vi "observacao.vi"() -> ()   [LabVIEW 2018, in "Shared_160.lvlib"] (continued)
                      }
                      frame True {
                        # "stop"
                      }
                    }
                  }
                  frame 3 {
                    w3458 = "TENTE NOVAMENTE" ("SYSTEM MESSAGES")
                    # "Trata Timeout"
                    n2721 = call "TickTimeout.vi"() -> ("msTick"=w3459:u32)  [unwired: 2 in, 2 out]
                    n2722 = call "Monta_Mensagem.vi"("Mensagem"=w3458) -> ()  [unwired: 2 in]
                    n2723 = call "Salva_systems_messages.vi"("Mensagem"=w3458) -> ()  [unwired: 5 in]
                    n2724 = local write "Timeout PROT"(w3459) -> ()
                  }
                  frame 4 {
                    w3462 = u16 1 items=["ZERO", "AH", "DEC", "TUBO", "CUP"] ("Controlador")
                    w3467 = u16 2 items=["ZERO", "AH", "DEC", "TUBO", "CUP"] ("Controlador")
                    # "Para os motores"
                    n2725 = call "Monta Comando.vi"("Comando"="PARAR", "Dispositivo"="PROG", "Controlador"=w3462) -> ()  [unwired: 2 in, 5 out]
                    n2726 = call "Monta Comando.vi"("Comando"="PARAR", "Dispositivo"="PROG", "Controlador"=w3467) -> ()  [unwired: 2 in, 5 out]
                  }
                  frame 5 {
                    # "SAÍDA"
                  }
                }
                n2727 = local write "M_PROT"(w3430) -> ()
              }
              frame #3 {
                w3486 = u16 3 items=["Alarme", "Atencao", "Erro", "Ocupado", "TBD", "LCB", "Trapeira", "Paravento", "DomoRap", "DomoCW", "DomoCCW", "TBD", "Em movimento", "TBD"] ("NomeStatus")
                w3492 = u16 3 items=["Alarme", "Atencao", "Erro", "Ocupado", "Protecao", "Embreagem", "Tracking", "Var. Track", "Rápido", "Ligeiro", "Médio", "Lento", "Em movimento", ""] ("NomeStatus")
                w3493 = u16 3 items=["Alarme", "Atencao", "Erro", "Ocupado", "Protecao", "Embreagem", "Tracking", "Var. Track", "Rápido", "Ligeiro", "Médio", "Lento", "Em movimento", ""] ("NomeStatus")
                n2728 = global read "Global_Telescopio.vi" "LimiarRapMed"() -> (w3494:dbl)
                n2729 = global read "Global_Telescopio.vi" "PosAH"() -> (w3496:dbl)
                n2730 = global read "Global_Telescopio.vi" "ErroMaxEixo"() -> (w3491:dbl)
                n2731 = global read "Global_Telescopio.vi" "PosDEC"() -> (w3495:dbl)
                n2732 = call "Bit Status DEC.vi"("NomeStatus"=w3492) -> ("StatBit"=w3490:bool)
                n2733 = call "Bit Status AH.vi"("NomeStatus"=w3493) -> ("StatBit"=w3489:bool)
                n2734 = case shown="3" "M_DEC" {
                  selector: "M_DEC" -> [w3588 _ _ _ _ _ _ _ _]
                  tunnel: [w3588 w3594 w3621 w3646 w3669 w3693 0 w3710 w3717] -> w3475
                  tunnel: "DestDEC" -> [_ w3593 w3618 w3640 w3666 _ _ _ w3727]
                  tunnel: w3495 -> [_ w3596 _ w3643 _ _ _ _ w3726]
                  tunnel: w3491 -> [_ _ _ w3644 _ _ _ _ _]
                  tunnel: w3494 -> [_ w3595 _ _ _ _ _ _ w3723]
                  tunnel: w3490 -> [_ w3592 _ w3639 _ _ _ _ _]
                  frame 0, Default {
                    w3586 = 0 ("CR DEC")
                    # "Sem apontamento"
                    n2735 = call "TickTimeout.vi"() -> ("msTick"=→"TimeoutDEC 2":u32)  [unwired: 2 in, 2 out]
                    "CR DEC UTILS" <- w3586
                    "CONT DEC UTILS" <- w3586
                  }
                  frame 1 {
                    # "Envia\nComando"
                    n2736 = Subtract(x=w3593, y=w3596) -> (x-y=w3591:dbl)
                    n2737 = Absolute Value(x=w3591) -> (abs(x)=w3597:dbl)
                    n2738 = Less?(x=w3597, y=w3595) -> (x < y?=w3590:bool)
                    n2739 = case shown="False" w3590 {
                      tunnel: [w3601 3] -> w3594
                      tunnel: w3593 -> [w3600 _]
                      tunnel: w3591 -> [w3599 _]
                      tunnel: w3592 -> [w3598 _]
                      frame False {
                        # "destino"
                        # "Fora do"
                        n2740 = case shown="False" w3598 {
                          tunnel: [20 w3610] -> w3601
                          tunnel: w3600 -> [w3604 _]
                          tunnel: w3599 -> [_ _]
                          frame False {
                            w3608 = u16 2 items=["ZERO", "AH", "DEC", "TUBO", "CUP"] ("Controlador")
                            # "CLP Pronto"
                            n2741 = local write "DEC on Target"(FALSE ("DEC on Target")) -> ()
                            n2742 = call "rad_hms.vi"("TRUE=HORA\nFALSE=GRAU"=FALSE, "Radiano"=w3604) -> ("Hora/Graus Texto Decimal"=w3605:string)  [unwired: 3 in]
                            n2743 = call "Monta Comando.vi"("Set Point"=w3605, "Comando"="MOVER_RAP", "Dispositivo"="EIXO" ("Comando"), "Controlador"=w3608) -> ()  [unwired: 1 in, 5 out]
                          }
                          frame True {
                            # "CLP Ocupado"
                            n2744 = local read "TimeoutDEC 2"() -> (w3612:u32)
                            n2745 = call "TickTimeout.vi"("msInicial"=w3612, "msTimeout"=u32 4000) -> ("Timeout"=w3611:bool)  [unwired: 2 out]
                            n2746 = case shown="False" w3611 {
                              tunnel: [1 5] -> w3610
                              frame False {
                              }
                              frame True {
                                # "Tratar\nTimeout"
                              }
                            }
                          }
                        }
                      }
                      frame True {
                        # "Dist. pequena p/ mov. rápido"
                        # "Ligar mov. lento"
                        n2747 = call "TickTimeout.vi"() -> ("msTick"=w3616:u32)  [unwired: 2 in, 2 out]
                        n2748 = local write "TimeoutDEC 2"(w3616) -> ()
                      }
                    }
                    n2749 = local write "dec="(FALSE ("dec=")) -> ()
                  }
                  frame 2 {
                    w3624 = u16 12 items=["Alarme", "Atencao", "Erro", "Ocupado", "Protecao", "Embreagem", "Tracking", "Var. Track", "Rápido", "Ligeiro", "Médio", "Lento", "Em movimento", ""] ("NomeStatus")
                    # "Aguarda fim mov. Rap."
                    n2750 = call "Bit Status DEC.vi"("NomeStatus"=w3624) -> ("StatBit"=w3625:bool)
                    n2751 = case shown="True" w3625 {
                      tunnel: [1 w3634] -> w3622
                      tunnel: w3618 -> [_ w3633]
                      frame False {
                        # "Motor parado.\nTestar se chegou\nao destino"
                        n2752 = call "TickTimeout.vi"() -> ("msTick"=w3630:u32)  [unwired: 2 in, 2 out]
                        n2753 = local write "TimeoutDEC 2"(w3630) -> ()
                      }
                      frame True {
                        # "Ainda movendo...\nAGUARDAR"
                        n2754 = call "PROTECAO_DEC_UTILS.vi"("Destino DEC"=w3633) -> ("CONT DEC"=w3632:i32)  [unwired: 10 in]
                        n2755 = local read "Erro PROTEC"() -> (w3635:i32)
                        n2756 = Greater Or Equal?(x=w3632, y=w3635) -> (x >= y?=w3638:bool)
                        n2757 = local write "CONT DEC UTILS"(w3632) -> ()
                        n2758 = Select(t=6, s=w3638, f=2) -> (s? t:f=w3634:i32)
                      }
                    }
                    n2759 = global read "Global_Telescopio.vi" "Habilita supervisao"() -> (w3620:bool)
                    n2760 = case shown="True" w3620 {
                      tunnel: [FALSE w3629] -> w3619
                      frame False {
                      }
                      frame True {
                        n2761 = local read "CR DEC UTILS"() -> (w3627:i32)
                        n2762 = local read "Erro Lim"() -> (w3628:i32)
                        n2763 = Greater Or Equal?(x=w3627, y=w3628) -> (x >= y?=w3629:bool)
                      }
                    }
                    n2764 = Select(t=6, s=w3619, f=w3622) -> (s? t:f=w3621:i32)
                  }
                  frame 3 {
                    # "Mov.Lento"
                    n2765 = Subtract(x=w3640, y=w3643) -> (x-y=w3641:dbl)
                    n2766 = Absolute Value(x=w3641) -> (abs(x)=w3645:dbl)
                    n2767 = Less Or Equal?(x=w3645, y=w3644) -> (x <= y?=w3642:bool)
                    n2768 = case shown="False" w3642 {
                      tunnel: [w3648 0] -> w3646
                      tunnel: w3641 -> [w3647 _]
                      tunnel: w3639 -> [w3649 _]
                      frame False {
                        n2769 = case shown="False" w3649 {
                          tunnel: [40 w3658] -> w3648
                          tunnel: w3647 -> [w3652 _]
                          frame False {
                            w3657 = u16 2 items=["ZERO", "AH", "DEC", "TUBO", "CUP"] ("Controlador")
                            # "Mov. lento"
                            n2770 = call "TickTimeout.vi"() -> ("msTick"=w3650:u32)  [unwired: 2 in, 2 out]
                            n2771 = local write "TimeoutDEC 2"(w3650) -> ()
                            n2772 = call "rad_hms.vi"("TRUE=HORA\nFALSE=GRAU"=FALSE ("TRUE=HORA\nFALSE=GRAU"), "Radiano"=w3652) -> ("Hora/Graus Texto Decimal"=w3654:string)  [unwired: 3 in]
                            n2773 = call "Monta Comando.vi"("Set Point"=w3654, "Comando"="MOVER_REL", "Dispositivo"="EIXO" ("Comando"), "Controlador"=w3657) -> ()  [unwired: 1 in, 5 out]
                          }
                          frame True {
                            # "CLP Ocupado"
                            n2774 = local read "TimeoutDEC 2"() -> (w3660:u32)
                            n2775 = call "TickTimeout.vi"("msInicial"=w3660, "msTimeout"=u32 2000) -> ("Timeout"=w3659:bool)  [unwired: 2 out]
                            n2776 = case shown="False" w3659 {
                              tunnel: [3 5] -> w3658
                              frame False {
                              }
                              frame True {
                              }
                            }
                          }
                        }
                      }
                      frame True {
                        # "DEC no destino"
                        n2777 = local write "DEC on Target"(TRUE ("DEC on Target")) -> ()
                      }
                    }
                  }
                  frame 4 {
                    w3672 = u16 12 items=["Alarme", "Atencao", "Erro", "Ocupado", "Protecao", "Embreagem", "Tracking", "Var. Track", "Rápido", "Ligeiro", "Médio", "Lento", "Em movimento", ""] ("NomeStatus")
                    # "Aguarda fim mov. lento"
                    n2778 = global read "Global_Telescopio.vi" "Habilita supervisao"() -> (w3671:bool)
                    n2779 = call "Bit Status DEC.vi"("NomeStatus"=w3672) -> ("StatBit"=w3673:bool)
                    n2780 = case shown="True" w3673 {
                      tunnel: [3 w3683] -> w3668
                      tunnel: w3666 -> [_ w3681]
                      frame False {
                        # "Motor parado.\nTestar se chegou\nao destino"
                        n2781 = call "TickTimeout.vi"() -> ("msTick"=w3678:u32)  [unwired: 2 in, 2 out]
                        n2782 = local write "TimeoutDEC 2"(w3678) -> ()
                      }
                      frame True {
                        n2783 = call "PROTECAO_DEC_UTILS.vi"("Destino DEC"=w3681) -> ("CONT DEC"=w3680:i32)  [unwired: 10 in]
                        n2784 = local read "Erro PROTEC"() -> (w3686:i32)
                        n2785 = local write "CONT DEC UTILS"(w3680) -> ()
                        n2786 = Greater Or Equal?(x=w3680, y=w3686) -> (x >= y?=w3688:bool)
                        n2787 = local read "TimeoutDEC 2"() -> (w3682:u32)
                        n2788 = call "TickTimeout.vi"("msInicial"=w3682, "msTimeout"=u32 4000) -> ("Timeout"=w3685:bool)  [unwired: 2 out]
                        n2789 = case shown="False" w3685 {
                          tunnel: [4 5] -> w3689
                          frame False {
                          }
                          frame True {
                          }
                        }
                        n2790 = Select(t=6, s=w3688, f=w3689) -> (s? t:f=w3683:i32)
                      }
                    }
                    n2791 = case shown="True" w3671 {
                      tunnel: [FALSE w3677] -> w3667
                      frame False {
                      }
                      frame True {
                        n2792 = local read "CR DEC UTILS"() -> (w3675:i32)
                        n2793 = local read "Erro Lim"() -> (w3676:i32)
                        n2794 = Greater Or Equal?(x=w3675, y=w3676) -> (x >= y?=w3677:bool)
                      }
                    }
                    n2795 = Select(t=6, s=w3667, f=w3668) -> (s? t:f=w3669:i32)
                  }
                  frame 5 {
                    w3699 = u16 2 items=["ZERO", "AH", "DEC", "TUBO", "CUP"] ("Controlador")
                    # "Reiniciar apontamento"
                    # "Trata Timeout"
                    n2796 = call "TickTimeout.vi"() -> ("msTick"=w3692:u32)  [unwired: 2 in, 2 out]
                    n2797 = local write "TimeoutDEC 2"(w3692) -> ()
                    n2798 = call "Monta Comando.vi"("Comando"="PARAR", "Dispositivo"="PROG" ("Comando"), "Controlador"=w3699) -> ("Erro Comunicação"=w3694:bool)  [unwired: 2 in, 4 out]
                    n2799 = Select(t=6, s=w3694, f=1) -> (s? t:f=w3693:i32)
                  }
                  frame 6 {
                    n2800 = stacked-sequence {
                      frame #0 {
                        w3704 = u16 2 items=["ZERO", "AH", "DEC", "TUBO", "CUP"] ("Controlador")
                        # "Trata Timeout"
                        n2801 = local write "dec="(TRUE ("dec=")) -> ()
                        n2802 = call "Monta Comando.vi"("Comando"="PARAR", "Dispositivo"="PROG" ("Comando"), "Controlador"=w3704) -> ()  [unwired: 2 in, 5 out]
                      }
                      frame #1 {
                        w3706 = "Erro de Controlador DEC , REAPONTAR !" ("Mensagem")
                        n2803 = local write "Flag de erro p/ apagar lampada"(TRUE ("Flag de erro p/ apagar lampada")) -> ()
                        n2804 = call "Monta_Mensagem.vi"("Mensagem"=w3706) -> ()  [unwired: 2 in]
                        n2805 = call "Salva_systems_messages.vi"("Mensagem"=w3706) -> ()  [unwired: 5 in]
                      }
                      frame #2 {
                        w3708 = u16 2 items=["ZERO", "AH", "DEC", "TUBO", "CUP"] ("Controlador")
                        # "Em movimento não aceita reset"
                        # "Segundo PARAR por garantia"
                        n2806 = call "Monta Comando.vi"("Comando"="PARAR", "Dispositivo"="PROG", "Controlador"=w3708) -> ()  [unwired: 2 in, 5 out]
                      }
                    }
                  }
                  frame 20 {
                    # "Espera entrar\nem movimento"
                    n2807 = local read "Flag ativo DEC"() -> (w3711:bool)
                    n2808 = case shown="True" w3711 {
                      tunnel: [20 ("t") 2 ("t")] -> w3710
                      frame False {
                      }
                      frame True {
                        # "limpa flag"
                        n2809 = local write "Flag ativo DEC"(FALSE ("Flag ativo AH")) -> ()
                      }
                    }
                  }
                  frame 40 {
                    # "INTERROMPE O\nMOVIMENTO"
                    # "Espera entrar\nem movimento"
                    n2810 = local read "TimeoutDEC 2"() -> (w3722:u32)
                    n2811 = Subtract(x=w3727, y=w3726) -> (x-y=w3725:dbl)
                    n2812 = local read "Flag ativo DEC"() -> (w3728:bool)
                    n2813 = Absolute Value(x=w3725) -> (abs(x)=w3724:dbl)
                    n2814 = call "TickTimeout.vi"("msInicial"=w3722, "msTimeout"=u32 2000) -> ("Timeout"=w3720:bool)  [unwired: 2 out]
                    n2815 = Less Or Equal?(x=w3724, y=w3723) -> (x <= y?=w3719:bool)
                    n2816 = case shown="True" w3728 {
                      tunnel: [40 ("t") 4 ("t")] -> w3718
                      frame False {
                      }
                      frame True {
                        # "limpa flag"
                        n2817 = local write "Flag ativo DEC"(FALSE ("Flag ativo AH")) -> ()
                      }
                    }
                    n2818 = Or(x=w3720, y=w3719) -> (x .or. y?=w3716:bool)
                    n2819 = Select(t=5, s=w3716, f=w3718) -> (s? t:f=w3717:i32)
                  }
                }
                n2820 = case shown="6" "M_AH" {
                  selector: "M_AH" -> [w3734 _ _ _ _ _ _ _ _ _ _]
                  tunnel: [w3734 w3735 w3755 w3786 5 w3809 w3838 w3860 0 w3878 w3883] -> w3477
                  tunnel: "DestAH" -> [_ _ w3752 w3782 _ w3805 w3834 _ _ _ _]
                  tunnel: w3496 -> [_ _ w3758 _ _ w3811 _ _ _ _ _]
                  tunnel: w3491 -> [_ _ _ _ _ w3810 _ _ _ _ _]
                  tunnel: w3494 -> [_ _ w3759 _ _ _ _ _ _ _ _]
                  tunnel: w3489 -> [_ w3736 w3753 _ _ w3807 _ _ _ _ _]
                  frame 0, Default {
                    w3732 = 0 ("CR AH")
                    # "Sem apontamento"
                    n2821 = call "TickTimeout.vi"() -> ("msTick"=→"TimeoutAH 2":u32)  [unwired: 2 in, 2 out]
                    "CR AH UTILS" <- w3732
                    "CONT AH UTILS" <- w3732
                  }
                  frame 1 {
                    n2822 = case shown="False" w3736 {
                      tunnel: [2 w3746] -> w3735
                      frame False {
                        n2823 = stacked-sequence {
                          frame #0 {
                            w3741 = u16 1 items=["ZERO", "AH", "DEC", "TUBO", "CUP"] ("Controlador")
                            # "Desliga Acomp Sideral"
                            n2824 = call "Monta Comando.vi"("Comando"="DESLIGAR", "Dispositivo"="SIDERAL" ("Comando"), "Controlador"=w3741) -> ()  [unwired: 2 in, 5 out]
                          }
                          frame #1 {
                            w3744 = u16 1 items=["ZERO", "AH", "DEC", "TUBO", "CUP"] ("Controlador")
                            # "Parar Eixo AH"
                            n2825 = call "Monta Comando.vi"("Comando"="PARAR", "Dispositivo"="PROG" ("Comando"), "Controlador"=w3744) -> ()  [unwired: 2 in, 5 out]
                          }
                        }
                        n2826 = call "TickTimeout.vi"() -> ("msTick"=w3737:u32)  [unwired: 2 in, 2 out]
                        n2827 = local write "TimeoutAH 2"(w3737) -> ()
                      }
                      frame True {
                        n2828 = local read "TimeoutAH 2"() -> (w3745:u32)
                        n2829 = call "TickTimeout.vi"("msInicial"=w3745, "msTimeout"=u32 5000) -> ("Timeout"=w3748:bool)  [unwired: 2 out]
                        n2830 = case shown="False" w3748 {
                          tunnel: [1 7] -> w3746
                          frame False {
                          }
                          frame True {
                          }
                        }
                      }
                    }
                  }
                  frame 2 {
                    # "Mov.Rapido"
                    n2831 = Subtract(x=w3752, y=w3758) -> (x-y=w3756:dbl)
                    n2832 = Absolute Value(x=w3756) -> (abs(x)=w3757:dbl)
                    n2833 = Less?(x=w3757, y=w3759) -> (x < y?=w3754:bool)
                    n2834 = case shown="False" w3754 {
                      tunnel: w3752 -> [w3760 _]
                      tunnel: w3756 -> [_ _]
                      tunnel: [w3761 4] -> w3755
                      tunnel: w3753 -> [w3762 _]
                      frame False {
                        n2835 = case shown="False" w3762 {
                          tunnel: w3760 -> [w3768 _]
                          tunnel: [w3763 w3774] -> w3761
                          frame False {
                            w3770 = u16 1 items=["ZERO", "AH", "DEC", "TUBO", "CUP"] ("Controlador")
                            # "Aguardar\nfim mov."
                            # "Mov. rápido"
                            n2836 = local write "RA on Target"(FALSE ("RA on Target")) -> ()
                            n2837 = call "rad_hms.vi"("TRUE=HORA\nFALSE=GRAU"=TRUE ("TRUE=HORA\nFALSE=GRAU"), "Radiano"=w3768) -> ("Hora/Graus Texto Decimal"=w3773:string)  [unwired: 3 in]
                            n2838 = call "Monta Comando.vi"("Set Point"=w3773, "Comando"="MOVER_RAP", "Dispositivo"="EIXO" ("Comando"), "Controlador"=w3770) -> ("Erro Comunicação"=w3764:bool)  [unwired: 1 in, 4 out]
                            n2839 = Select(t=8, s=w3764, f=30) -> (s? t:f=w3763:i32)
                          }
                          frame True {
                            # "CLP Ocupado"
                            n2840 = local read "TimeoutAH 2"() -> (w3776:u32)
                            n2841 = call "TickTimeout.vi"("msInicial"=w3776, "msTimeout"=u32 4000) -> ("Timeout"=w3775:bool)  [unwired: 2 out]
                            n2842 = case shown="True" w3775 {
                              tunnel: [2 7] -> w3774
                              frame False {
                              }
                              frame True {
                                # "Tratar\nTimeout"
                              }
                            }
                          }
                        }
                      }
                      frame True {
                        # "Dist. pequena p/ mov. rápido"
                        n2843 = call "TickTimeout.vi"() -> ("msTick"=w3780:u32)  [unwired: 2 in, 2 out]
                        n2844 = local write "TimeoutAH 2"(w3780) -> ()
                      }
                    }
                    n2845 = local write "ah="(FALSE ("ah=")) -> ()
                  }
                  frame 3 {
                    w3789 = u16 12 items=["Alarme", "Atencao", "Erro", "Ocupado", "Protecao", "Embreagem", "Tracking", "Var. Track", "Rápido", "Ligeiro", "Médio", "Lento", "Em movimento", ""] ("NomeStatus")
                    # "Aguarda fim mov. Rap."
                    n2846 = call "Bit Status AH.vi"("NomeStatus"=w3789) -> ("StatBit"=w3788:bool)
                    n2847 = case shown="True" w3788 {
                      tunnel: [2 w3798] -> w3785
                      tunnel: w3782 -> [_ w3797]
                      frame False {
                        # "Motor parado.\nTestar se precisa\nde novo cmd. \nde mov. rápido"
                        n2848 = call "TickTimeout.vi"() -> ("msTick"=w3794:u32)  [unwired: 2 in, 2 out]
                        n2849 = local write "TimeoutAH 2"(w3794) -> ()
                      }
                      frame True {
                        # "Aqui também \ncaberia um \nTimeout?"
                        # "Ainda movendo...\nAGUARDAR"
                        n2850 = call "PROTECAO_AH_UTILS.vi"("DestinoAH"=w3797) -> ("CONT AH"=w3796:i32)  [unwired: 10 in]
                        n2851 = local read "Erro PROTEC"() -> (w3800:i32)
                        n2852 = local write "CONT AH UTILS"(w3796) -> ()
                        n2853 = Greater Or Equal?(x=w3796, y=w3800) -> (x >= y?=w3801:bool)
                        n2854 = Select(t=8, s=w3801, f=3) -> (s? t:f=w3798:i32)
                      }
                    }
                    n2855 = global read "Global_Telescopio.vi" "Habilita supervisao"() -> (w3784:bool)
                    n2856 = case shown="True" w3784 {
                      tunnel: [FALSE w3793] -> w3783
                      frame False {
                      }
                      frame True {
                        n2857 = local read "Erro Lim"() -> (w3792:i32)
                        n2858 = local read "CR AH UTILS"() -> (w3791:i32)
                        n2859 = Greater Or Equal?(x=w3791, y=w3792) -> (x >= y?=w3793:bool)
                      }
                    }
                    n2860 = Select(t=8, s=w3783, f=w3785) -> (s? t:f=w3786:i32)
                  }
                  frame 4 {
                    # "Não faz nada"
                    n2861 = call "TickTimeout.vi"() -> ("msTick"=w3804:u32)  [unwired: 2 in, 2 out]
                    n2862 = local write "TimeoutAH 2"(w3804) -> ()
                  }
                  frame 5 {
                    # "Mov.Lento"
                    n2863 = Subtract(x=w3805, y=w3811) -> (x-y=w3806:dbl)
                    n2864 = Absolute Value(x=w3806) -> (abs(x)=w3812:dbl)
                    n2865 = Less Or Equal?(x=w3812, y=w3810) -> (x <= y?=w3808:bool)
                    n2866 = case shown="True" w3808 {
                      tunnel: w3806 -> [w3814 _]
                      tunnel: [w3813 0] -> w3809
                      tunnel: w3807 -> [w3815 _]
                      frame False {
                        n2867 = case shown="False" w3815 {
                          tunnel: w3814 -> [w3820 _]
                          tunnel: [w3819 w3826] -> w3813
                          frame False {
                            w3822 = u16 1 items=["ZERO", "AH", "DEC", "TUBO", "CUP"] ("Controlador")
                            # "Envia Cmd. Mov. Lento"
                            n2868 = call "rad_hms.vi"("TRUE=HORA\nFALSE=GRAU"=TRUE ("TRUE=HORA\nFALSE=GRAU"), "Radiano"=w3820) -> ("Hora/Graus Texto Decimal"=w3825:string)  [unwired: 3 in]
                            n2869 = call "Monta Comando.vi"("Set Point"=w3825, "Comando"="MOVER_REL", "Dispositivo"="EIXO" ("Comando"), "Controlador"=w3822) -> ("Erro Comunicação"=w3817:bool)  [unwired: 1 in, 4 out]
                            n2870 = Select(t=8, s=w3817, f=60) -> (s? t:f=w3819:i32)
                          }
                          frame True {
                            # "CLP Ocupado"
                            n2871 = local read "TimeoutAH 2"() -> (w3828:u32)
                            n2872 = call "TickTimeout.vi"("msInicial"=w3828, "msTimeout"=u32 4000) -> ("Timeout"=w3827:bool)  [unwired: 2 out]
                            n2873 = case shown="False" w3827 {
                              tunnel: [5 7] -> w3826
                              frame False {
                              }
                              frame True {
                              }
                            }
                          }
                        }
                      }
                      frame True {
                        # "AH on Target"
                        n2874 = local write "RA on Target"(TRUE ("RA on Target")) -> ()
                      }
                    }
                  }
                  frame 6 {
                    w3841 = u16 12 items=["Alarme", "Atencao", "Erro", "Ocupado", "Protecao", "Embreagem", "Tracking", "Var. Track", "Rápido", "Ligeiro", "Médio", "Lento", "Em movimento", ""] ("NomeStatus")
                    # "Aguarda fim mov. Lento"
                    n2875 = call "Bit Status AH.vi"("NomeStatus"=w3841) -> ("StatBit"=w3840:bool)
                    n2876 = case shown="True" w3840 {
                      tunnel: [5 w3855] -> w3837
                      tunnel: w3834 -> [_ w3849]
                      frame False {
                        # "Motor parado.\nTestar se chegou\nao destino"
                        n2877 = call "TickTimeout.vi"() -> ("msTick"=w3846:u32)  [unwired: 2 in, 2 out]
                        n2878 = local write "TimeoutAH 2"(w3846) -> ()
                      }
                      frame True {
                        n2879 = local read "Erro PROTEC"() -> (w3857:i32)
                        n2880 = call "PROTECAO_AH_UTILS.vi"("DestinoAH"=w3849) -> ("CONT AH"=w3848:i32)  [unwired: 10 in]
                        n2881 = local write "CONT AH UTILS"(w3848) -> ()
                        n2882 = local read "TimeoutAH 2"() -> (w3850:u32)
                        n2883 = Greater Or Equal?(x=w3848, y=w3857) -> (x >= y?=w3851:bool)
                        n2884 = call "TickTimeout.vi"("msInicial"=w3850, "msTimeout"=u32 4000) -> ("Timeout"=w3854:bool)  [unwired: 2 out]
                        n2885 = case shown="False" w3854 {
                          tunnel: [6 7] -> w3852
                          frame False {
                          }
                          frame True {
                            # "Tratar\nTimeout"
                          }
                        }
                        n2886 = Select(t=8, s=w3851, f=w3852) -> (s? t:f=w3855:i32)
                      }
                    }
                    n2887 = global read "Global_Telescopio.vi" "Habilita supervisao"() -> (w3836:bool)
                    n2888 = case shown="True" w3836 {
                      tunnel: [FALSE w3845] -> w3835
                      frame False {
                      }
                      frame True {
                        n2889 = local read "CR AH UTILS"() -> (w3843:i32)
                        n2890 = local read "Erro Lim"() -> (w3844:i32)
                        n2891 = Greater Or Equal?(x=w3843, y=w3844) -> (x >= y?=w3845:bool)
                      }
                    }
                    n2892 = Select(t=8, s=w3835, f=w3837) -> (s? t:f=w3838:i32)
                  }
                  frame 7 {
                    w3865 = u16 1 items=["ZERO", "AH", "DEC", "TUBO", "CUP"] ("Controlador")
                    # "Reiniciar apontamento"
                    # "Trata Timeout"
                    n2893 = call "TickTimeout.vi"() -> ("msTick"=w3864:u32)  [unwired: 2 in, 2 out]
                    n2894 = local write "TimeoutAH 2"(w3864) -> ()
                    n2895 = call "Monta Comando.vi"("Comando"="PARAR", "Dispositivo"="PROG" ("Comando"), "Controlador"=w3865) -> ("Erro Comunicação"=w3861:bool)  [unwired: 2 in, 4 out]
                    n2896 = Select(t=8, s=w3861, f=2) -> (s? t:f=w3860:i32)
                  }
                  frame 8 {
                    n2897 = stacked-sequence {
                      frame #0 {
                        w3870 = u16 1 items=["ZERO", "AH", "DEC", "TUBO", "CUP"] ("Controlador")
                        # "Reiniciar apontamento"
                        # "Trata Timeout"
                        n2898 = local write "ah="(TRUE ("ah=")) -> ()
                        n2899 = call "Monta Comando.vi"("Comando"="PARAR", "Dispositivo"="PROG" ("Comando"), "Controlador"=w3870) -> ()  [unwired: 2 in, 5 out]
                      }
                      frame #1 {
                        w3874 = "Erro de Controlador RA , REAPONTAR !" ("Mensagem")
                        n2900 = local write "Flag de erro p/ apagar lampada"(TRUE ("Flag de erro p/ apagar lampada")) -> ()
                        n2901 = call "Monta_Mensagem.vi"("Mensagem"=w3874) -> ()  [unwired: 2 in]
                        n2902 = call "Salva_systems_messages.vi"("Mensagem"=w3874) -> ()  [unwired: 5 in]
                      }
                      frame #2 {
                        w3877 = u16 1 items=["ZERO", "AH", "DEC", "TUBO", "CUP"] ("Controlador")
                        # "Em movimento não aceita reset"
                        # "Segundo PARAR por garantia"
                        n2903 = call "Monta Comando.vi"("Comando"="PARAR", "Dispositivo"="PROG", "Controlador"=w3877) -> ()  [unwired: 2 in, 5 out]
                      }
                    }
                  }
                  frame 30 {
                    # "Espera entrar\nem movimento"
                    n2904 = local read "Flag ativo AH"() -> (w3879:bool)
                    n2905 = case shown="True" w3879 {
                      tunnel: [30 ("t") 3 ("t")] -> w3878
                      frame False {
                      }
                      frame True {
                        # "limpa flag"
                        n2906 = local write "Flag ativo AH"(FALSE ("Flag ativo AH")) -> ()
                      }
                    }
                  }
                  frame 60 {
                    # "Espera entrar\nem movimento"
                    n2907 = local read "Flag ativo AH"() -> (w3884:bool)
                    n2908 = case shown="True" w3884 {
                      tunnel: [60 ("t") 6 ("t")] -> w3883
                      frame False {
                      }
                      frame True {
                        # "limpa flag"
                        n2909 = local write "Flag ativo AH"(FALSE ("Flag ativo AH")) -> ()
                      }
                    }
                  }
                }
                n2910 = call "PROTECAO.vi"("Estado In"=w3477) -> ("Estado Out"=w3476:i32)  [unwired: 2 in]
                n2911 = call "PROTECAO.vi"("Estado In"=w3475) -> ("Estado Out"=w3474:i32)  [unwired: 2 in]
                n2912 = local read "M_PROT"() -> (w3471:i32)
                n2913 = property on="Setup, Pointing & Guiding" class="TabCtl (strict)"() -> ("Page Selector Visible"=w3481:bool)  [unwired: 2 in, 2 out]
                n2914 = call "Bit Status CUP.vi"("NomeStatus"=w3486) -> ("StatBit"=w3488:bool)
                n2915 = local write "M_DEC"(w3474) -> ()
                n2916 = Not(x=w3481) -> (.not. x?=w3479:bool)
                n2917 = case shown="5" "M_CUP" {
                  selector: "M_CUP" -> [w3501 _ _ _ _ _ _ _ _]
                  tunnel: [w3501 w3506 w3533 1 w3544 w3557 w3562 w3579 0 ("estadoCUP")] -> w3473
                  tunnel: w3488 -> [_ w3507 _ _ w3543 _ w3563 _ _]
                  tunnel: "DestCUP" -> [_ w3505 _ _ _ _ _ _ _]
                  frame 0, Default {
                    # "Sem movimento"
                    n2918 = call "TickTimeout.vi"() -> ("msTick"=→"TimeoutCUP 2":u32)  [unwired: 2 in, 2 out]
                  }
                  frame 1 {
                    # "20240820"
                    # "Envia\nComando"
                    n2919 = call "Checa destino cupula.vi"("Target"=w3505) -> ("moverCup"=w3504:bool, "angTarget"=w3502:string)  [unwired: 6 in, 1 out]
                    n2920 = Not(x=w3504) -> (.not. x?=w3503:bool)
                    n2921 = case shown="True" w3503 {
                      tunnel: w3507 -> [w3511 _]
                      tunnel: w3505 -> [w3510 _]
                      tunnel: [w3509 w3527] -> w3506
                      tunnel: w3502 -> [w3508 _]
                      frame False {
                        # "CUP fora pos."
                        n2922 = case shown="False" w3511 {
                          tunnel: w3510 -> [w3520 _]
                          tunnel: [2 w3521] -> w3509
                          tunnel: w3508 -> [w3512 _]
                          frame False {
                            w3517 = u16 4 items=["ZERO", "AH", "DEC", "TUBO", "CUP"] ("Controlador")
                            # "CLP Pronto"
                            n2923 = call "TickTimeout.vi"() -> ("msTick"=w3516:u32)  [unwired: 2 in, 2 out]
                            n2924 = Number To Decimal String(number=w3520) -> (decimal integer string=w3513:string)  [unwired: 1 in]
                            n2925 = local write "TimeoutCUP 2"(w3516) -> ()
                            n2926 = local write "Dome on Target"(FALSE ("Dome on Target")) -> ()
                            n2927 = local write "TargetCup"(w3512) -> ()
                            n2928 = call "Monta Comando.vi"("Set Point"=w3513, "Comando"="MOVER", "Dispositivo"="DOMO" ("Comando"), "Controlador"=w3517) -> ()  [unwired: 1 in, 5 out]
                          }
                          frame True {
                            # "CLP Busy"
                            n2929 = local read "TimeoutCUP 2"() -> (w3523:u32)
                            n2930 = call "TickTimeout.vi"("msInicial"=w3523, "msTimeout"=u32 5000) -> ("Timeout"=w3522:bool)  [unwired: 2 out]
                            n2931 = case shown="True" w3522 {
                              tunnel: [1 3] -> w3521
                              frame False {
                              }
                              frame True {
                              }
                            }
                          }
                        }
                      }
                      frame True {
                        # "Verifica\nTrapeira e\nParavento"
                        # "CUP no destino"
                        n2932 = call "TickTimeout.vi"() -> ("msTick"=w3531:u32)  [unwired: 2 in, 2 out]
                        n2933 = global read "Global_Telescopio.vi" "Parking"() -> (w3530:bool)
                        n2934 = local write "TimeoutCUP 2"(w3531) -> ()
                        n2935 = Select(t=4, s=w3530, f=8) -> (s? t:f=w3527:i32)
                      }
                    }
                  }
                  frame 2 {
                    w3532 = u16 12 items=["Alarme", "Atencao", "Erro", "Ocupado", "TBD", "LCB", "Trapeira", "Paravento", "DomoRap", "DomoCW", "DomoCCW", "TBD", "Em movimento", "TBD"] ("NomeStatus")
                    # "Aqui também caberia um Timeout?"
                    # "Aguarda parada motor"
                    n2936 = call "Bit Status CUP.vi"("NomeStatus"=w3532) -> ("StatBit"=w3534:bool)
                    n2937 = case shown="True" w3534 {
                      tunnel: [1 2] -> w3533
                      frame False {
                        # "Motor parado.\nTestar se chegou\nao destino"
                        n2938 = call "TickTimeout.vi"() -> ("msTick"=w3535:u32)  [unwired: 2 in, 2 out]
                        n2939 = local write "TimeoutCUP 2"(w3535) -> ()
                      }
                      frame True {
                        # "Ainda movendo...\nAGUARDAR"
                      }
                    }
                  }
                  frame 3 {
                    w3541 = u16 4 items=["ZERO", "AH", "DEC", "TUBO", "CUP"] ("Controlador")
                    # "Trata Timeout"
                    n2940 = call "TickTimeout.vi"() -> ("msTick"=w3538:u32)  [unwired: 2 in, 2 out]
                    n2941 = local write "TimeoutCUP 2"(w3538) -> ()
                    n2942 = call "Monta Comando.vi"("Comando"="PARAR", "Dispositivo"="PROG" ("Comando"), "Controlador"=w3541) -> ()  [unwired: 2 in, 5 out]
                  }
                  frame 4 {
                    # "Verifica Trapeira"
                    n2943 = case shown="False" w3543 {
                      tunnel: [5 w3549] -> w3544
                      frame False {
                        w3548 = u16 4 items=["ZERO", "AH", "DEC", "TUBO", "CUP"] ("Controlador")
                        # "Fechar Trapeira"
                        # "Aguardar abertura Trap."
                        # "CLP Pronto"
                        n2944 = call "Monta Comando.vi"("Comando"="FECHAR", "Dispositivo"="TRAPEIRA" ("Comando"), "Controlador"=w3548) -> ()  [unwired: 2 in, 5 out]
                      }
                      frame True {
                        # "CLP Busy"
                        n2945 = local read "TimeoutCUP 2"() -> (w3551:u32)
                        n2946 = call "TickTimeout.vi"("msInicial"=w3551, "msTimeout"=u32 5000) -> ("Timeout"=w3550:bool)  [unwired: 2 out]
                        n2947 = case shown="False" w3550 {
                          tunnel: [4 3] -> w3549
                          frame False {
                          }
                          frame True {
                          }
                        }
                      }
                    }
                  }
                  frame 5 {
                    w3556 = u16 14 items=["Alarme", "Atencao", "Erro", "Ocupado", "Plataforma", "LCB", "Trapeira", "Paravento", "DomoRap", "DomoCW", "DomoCCW", "TBD", "Em movimento", "TrapRUN", "TrapFCH", "TrapABT"] ("NomeStatus")
                    # "Aqui também caberia um Timeout?"
                    # "Aguarda Fechamento da Trapeira"
                    n2948 = call "Bit Status CUP.vi"("NomeStatus"=w3556) -> ("StatBit"=w3555:bool)
                    n2949 = case shown="True" w3555 {
                      tunnel: [5 6] -> w3557
                      frame False {
                        # "Ainda movendo...\nAGUARDAR"
                      }
                      frame True {
                        # "Trapeira Fechada.\nVerificar Paravento."
                        n2950 = call "TickTimeout.vi"() -> ("msTick"=w3559:u32)  [unwired: 2 in, 2 out]
                        n2951 = local write "TimeoutCUP 2"(w3559) -> ()
                      }
                    }
                  }
                  frame 6 {
                    # "Verifica Paravento"
                    n2952 = case shown="True" "Case Ct" {
                      tunnel: w3563 -> [_ w3566]
                      tunnel: [8 w3565] -> w3562
                      frame False {
                        # "Paravento Elevado"
                      }
                      frame True {
                        # "Subir Parav."
                        n2953 = case shown="True" w3566 {
                          tunnel: [7 w3571] -> w3565
                          frame False {
                            w3570 = u16 4 items=["ZERO", "AH", "DEC", "TUBO", "CUP"] ("Controlador")
                            # "Aguardar subida Parav."
                            # "CLP Pronto"
                            n2954 = call "Monta Comando.vi"("Comando"="SUBIR", "Dispositivo"="PARAVENTO" ("Comando"), "Controlador"=w3570) -> ()  [unwired: 2 in, 5 out]
                          }
                          frame True {
                            # "CLP Busy"
                            n2955 = local read "TimeoutCUP 2"() -> (w3573:u32)
                            n2956 = call "TickTimeout.vi"("msInicial"=w3573, "msTimeout"=u32 5000) -> ("Timeout"=w3572:bool)  [unwired: 2 out]
                            n2957 = case shown="True" w3572 {
                              tunnel: [6 3] -> w3571
                              frame False {
                              }
                              frame True {
                              }
                            }
                          }
                        }
                      }
                    }
                  }
                  frame 7 {
                    w3578 = u16 7 items=["Alarme", "Atencao", "Erro", "Ocupado", "TBD", "LCB", "Trapeira", "Paravento", "DomoRap", "DomoCW", "DomoCCW", "TBD", "Em movimento", "TBD"] ("NomeStatus")
                    # "Também poderia ser testado o bit \"Em movimento\".\nNeste caso o código do \"IF\" deve ser permutado."
                    # "Aguarda Subida Paravento"
                    n2958 = call "Bit Status CUP.vi"("NomeStatus"=w3578) -> ("StatBit"=w3580:bool)
                    n2959 = Not(x=w3580) -> (.not. x?=w3577:bool)
                    n2960 = case shown="False" w3577 {
                      tunnel: [7 8] -> w3579
                      frame False {
                        # "Ainda movendo...\nAGUARDAR"
                      }
                      frame True {
                        # "Paravento elevado."
                      }
                    }
                  }
                  frame 8 {
                    # "CUP on target"
                    n2961 = local write "Dome on Target"(TRUE ("Dome on Target")) -> ()
                    n2962 = global write "Global_Telescopio.vi" "Parking"(FALSE) -> ()
                  }
                }
                n2963 = call "PROTECAO.vi"("Estado In"=w3473) -> ("Estado Out"=w3472:i32)  [unwired: 2 in]
                n2964 = Compound Arithmetic op=ADD(w3471, w3472, w3476, w3474) -> (w3482:i32)
                n2965 = Equal To 0?(x=w3482) -> (x = 0?=w3480:bool)
                n2966 = And(x=w3480, y=w3479) -> (x .and. y?=w3478:bool)
                n2967 = case shown="True" w3478 {
                  frame False {
                  }
                  frame True {
                    w3497 = FALSE
                    w3498 = u8 0 ("Disabled")
                    # "DESLIGA TODOS"
                    # "HABILITA TODOS"
                    n2968 = local write "BtUtilZenith"(w3497) -> ()
                    n2969 = local write "BtUtilPark"(w3497) -> ()
                    n2970 = local write "PROTEÇÃO"(w3497) -> ()
                    n2971 = local write "FLAT-FIELD"(w3497) -> ()
                    n2972 = local write "ECASS"(w3497) -> ()
                    n2973 = property on="BtUtilPark" class="Bool (strict)"("Disabled"=w3498) -> ()  [unwired: 2 in, 2 out]
                    n2974 = property on="ECASS" class="Bool (strict)"("Disabled"=w3498) -> ()  [unwired: 2 in, 2 out]
                    n2975 = property on="Setup, Pointing & Guiding" class="TabCtl (strict)"("Page Selector Visible"=TRUE) -> ()  [unwired: 2 in, 2 out]
                    n2976 = property on="BtUtilZenith" class="Bool (strict)"("Disabled"=w3498) -> ()  [unwired: 2 in, 2 out]
                    n2977 = property on="FLAT-FIELD" class="Bool (strict)"("Disabled"=w3498) -> ()  [unwired: 2 in, 2 out]
                    n2978 = property on="PROTEÇÃO" class="Bool (strict)"("Disabled"=w3498) -> ()  [unwired: 2 in, 2 out]
                  }
                }
                n2979 = local write "M_AH"(w3476) -> ()
                n2980 = local write "M_CUP"(w3472) -> ()
              }
              frame #4 {
                n2981 = case shown="True" "GO" {
                  frame False {
                  }
                  frame True {
                    w3892 = u16 3 items=["Alarme", "Atencao", "Erro", "Ocupado", "Protecao", "Embreagem", "Tracking", "Var. Track", "Rápido", "Ligeiro", "Médio", "Lento", "Em movimento", ""] ("NomeStatus")
                    w3893 = u16 3 items=["Alarme", "Atencao", "Erro", "Ocupado", "Protecao", "Embreagem", "Tracking", "Var. Track", "Rápido", "Ligeiro", "Médio", "Lento", "Em movimento", ""] ("NomeStatus")
                    n2982 = call "Bit Status AH.vi"("NomeStatus"=w3893) -> ("StatBit"=w3891:bool)
                    n2983 = call "Bit Status DEC.vi"("NomeStatus"=w3892) -> ("StatBit"=w3890:bool)
                    n2984 = Or(x=w3891, y=w3890) -> (x .or. y?=w3889:bool)
                    n2985 = case shown="False" w3889 {
                      frame False {
                        w3894 = FALSE ("RA on Target")
                        w3912 = u16 1 items=["ZERO", "AH", "DEC", "TUBO", "CUP"] ("Controlador")
                        w3917 = u16 2 items=["ZERO", "AH", "DEC", "TUBO", "CUP"] ("Controlador")
                        w3895 = FALSE ("GO")
                        n2986 = local write "RA on Target"(w3894) -> ()
                        n2987 = local write "DEC on Target"(w3894) -> ()
                        n2988 = global read "Global_Telescopio.vi" "Calagem AH"() -> (w3905:dbl)
                        n2989 = call "Comma_to_Point.vi"("Lat_A"="StrPointObjRA 2") -> ("Saída"=w3899:string)
                        n2990 = call "Comma_to_Point.vi"("Lat_A"="StrPointObjDEC 2") -> ("Saída"=w3896:string)
                        n2991 = global read "Global_Telescopio.vi" "Calagem DEC"() -> (w3904:dbl)
                        n2992 = call "hms_rad.vi"("True = hora"=TRUE, "Texto Graus"=w3899) -> ("radianos"=w3900:dbl)  [unwired: 3 in]
                        n2993 = call "hms_rad.vi"("True = hora"=FALSE, "Texto Graus"=w3896) -> ("radianos"=w3901:dbl)  [unwired: 3 in]
                        n2994 = Add(x=w3900, y=w3905) -> (x+y=w3903:dbl)
                        n2995 = Add(x=w3901, y=w3904) -> (x+y=w3902:dbl)
                        n2996 = local write "GO"(w3895) -> ()
                        n2997 = global write "Global_Telescopio.vi" "ObjCentrado"(w3895) -> ()
                        n2998 = call "rad_hms.vi"("TRUE=HORA\nFALSE=GRAU"=TRUE ("TRUE=HORA\nFALSE=GRAU"), "Radiano"=w3903) -> ("Hora/Graus Texto Decimal"=w3909:string)  [unwired: 3 in]
                        n2999 = call "rad_hms.vi"("TRUE=HORA\nFALSE=GRAU"=FALSE, "Radiano"=w3902) -> ("Hora/Graus Texto Decimal"=w3908:string)  [unwired: 3 in]
                        n3000 = call "Monta Comando.vi"("Set Point"=w3909, "Comando"="MOVER_ABS", "Dispositivo"="EIXO" ("Comando"), "Controlador"=w3912) -> ()  [unwired: 1 in, 5 out]
                        n3001 = call "Monta Comando.vi"("Set Point"=w3908, "Comando"="MOVER_ABS", "Dispositivo"="EIXO" ("Comando"), "Controlador"=w3917) -> ()  [unwired: 1 in, 5 out]
                      }
                      frame True {
                      }
                    }
                  }
                }
              }
            }
          }
        }
      }
      frame #3 {
        # "Desabiita Centragem\ndurante apontamento"
        # "PROCESSO TRACKING"
        # "Comando Via serial do Sistema de Aquisição"
        # "CHAVES PAINEL"
        n3002 = case shown="True" "BtShutterClose" {
          frame False {
          }
          frame True {
            w3961 = u16 3 items=["Alarme", "Atencao", "Erro", "Ocupado", "TBD", "LCB", "Trapeira", "Paravento", "DomoRap", "DomoCW", "DomoCCW", "TBD", "Em movimento", "TBD"] ("NomeStatus")
            n3003 = call "Bit Status CUP.vi"("NomeStatus"=w3961) -> ("StatBit"=w3962:bool)
            n3004 = case shown="False" w3962 {
              selector: w3962 -> [w3963 _]
              frame False {
                w3966 = u16 4 items=["ZERO", "AH", "DEC", "TUBO", "CUP"] ("Controlador")
                n3005 = local write "BtShutterClose"(w3963) -> ()
                n3006 = call "Monta Comando.vi"("Comando"="FECHAR", "Dispositivo"="TRAPEIRA" ("Comando"), "Controlador"=w3966) -> ()  [unwired: 2 in, 5 out]
              }
              frame True {
              }
            }
          }
        }
        n3007 = case shown="True" "Stop All" {
          frame False {
          }
          frame True {
            # "MUDANÇA:\nDesligada chave do\nacompanhamento."
            n3008 = local write "MOUNT"(FALSE ("Led Start/Stop")) -> ()
            n3009 = global write "Global_Telescopio.vi" "STOP ALL"(TRUE ("STOP ALL")) -> ()
          }
        }
        n3010 = control-ref of="BtTargetPoint"() -> (w3925:refnum<vi>)
        n3011 = case shown="True" "STOP" {
          frame False {
          }
          frame True {
            n3012 = stacked-sequence {
              frame #0 {
                n3013 = call "Stop.vi"() -> ()  [unwired: 1 in, 1 out]
              }
              frame #1 {
                w3955 = 0 ("estado")
                n3014 = local write "statDEC"(w3955) -> ()
                n3015 = local write "statAH"(w3955) -> ()
                n3016 = local write "statCUP"(w3955) -> ()
              }
              frame #2 {
                w3956 = 0 ("estado")
                n3017 = local write "M_AH"(w3956) -> ()
                n3018 = local write "M_DEC"(w3956) -> ()
                n3019 = local write "M_CUP"(w3956) -> ()
                n3020 = local write "M_PROT"(w3956) -> ()
              }
              frame #3 {
                w3957 = FALSE
                n3021 = local write "BtUtilZenith"(w3957) -> ()
                n3022 = local write "BtUtilPark"(w3957) -> ()
                n3023 = local write "FLAT-FIELD"(w3957) -> ()
                n3024 = local write "ECASS"(w3957) -> ()
                n3025 = local write "PROTEÇÃO"(w3957) -> ()
              }
              frame #4 {
                n3026 = case shown="True" "LedPointing" {
                  frame False {
                  }
                  frame True {
                    n3027 = local write "LedPointing"(FALSE ("LedPointing")) -> ()
                    n3028 = global write "Global_Telescopio.vi" "Botão GO = STOP"(TRUE ("Botão GO = STOP")) -> ()
                  }
                }
              }
            }
          }
        }
        n3029 = global read "Global_Telescopio.vi" "Centragem Via Aquisicao"() -> (w3932:bool)
        n3030 = property class="Bool"(reference=w3925) -> ("Boolean Text.Text"=w3926:string)  [unwired: 1 in, 2 out]
        n3031 = And(x="Enable Centragem", y=w3932) -> (x .and. y?=w3931:bool)
        n3032 = Or(x="BtOnTatget", y=w3931) -> (x .or. y?=w3928:bool)
        n3033 = local read "FLAT-FIELD"() -> (w3918:bool)
        n3034 = local read "BtUtilZenith"() -> (w3919:bool)
        n3035 = Equal?(x=w3926, y="STOP") -> (x = y?=w3924:bool)
        n3036 = Not(x=w3924) -> (.not. x?=w3923:bool)
        n3037 = And(x=w3923, y=w3928) -> (x .and. y?=w3929:bool)
        n3038 = Or(x=w3919, y=w3918) -> (x .or. y?=w3920:bool)
        n3039 = case shown="True" w3929 {
          frame False {
          }
          frame True {
            n3040 = stacked-sequence {
              seq-local: [w3967 _ _ _ _] -> [_ _ _ _ w4080]
              seq-local: [_ w3981 _ _ _] -> [_ _ _ _ w4081]
              seq-local: [_ _ w3995 _ _] -> [_ _ _ _ w4082]
              seq-local: [_ _ _ w4028 _] -> [_ _ _ _ w4059]
              frame #0 {
                # "Transforma estados lógicos\nnuma string hexadecimal"
                n3041 = local read "Processa Centragem"() -> (w3971:bool)
                n3042 = local read "MOV_IDX_AH"() -> (w3969:bool)
                n3043 = local read "ChkModel"() -> (w3973:bool)
                n3044 = local read "MOV_IDX_DEC"() -> (w3968:bool)
                n3045 = global read "Global_Telescopio.vi" "CalLocal"() -> (w3975:bool)
                n3046 = global read "Global_Telescopio.vi" "CalGlobal"() -> (w3974:bool)
                n3047 = global read "Global_Telescopio.vi" "CoordDia"() -> (w3972:bool)
                n3048 = global read "Global_Telescopio.vi" "ObjCentrado"() -> (w3970:bool)
                n3049 = Build Array(w3975, w3974, w3973, w3972, w3971, w3970, w3969, w3968) -> (w3978:bool[])
                n3050 = Boolean Array To Number(Boolean array=w3978) -> (number=w3977:u32)
                n3051 = Number To Hexadecimal String(1:i16 2 ("width (-)"), 2:w3977) -> (0:w3967:string)
              }
              frame #1 {
                w3982 = "\t"
                # "Reseta Flag do comando oriundo\nda comunicação serial Aquisição"
                n3052 = local read "ChkPointPrecessed"() -> (w3979:bool)
                n3053 = local read "StrPointObjName"() -> (w3985:string)
                "NAME" <- w3985
                n3054 = local read "StrPointObjRA"() -> (w3984:string)
                "RA" <- w3984
                n3055 = local read "StrPointObjDEC"() -> (w3983:string)
                "DEC" <- w3983
                n3056 = case shown="True" w3979 {
                  tunnel: ["2000.000000000" ("Saída") w3989] -> w3980
                  frame False {
                  }
                  frame True {
                    # "20240805"
                    n3057 = call "Calcula epoch.vi"() -> ("epoch"=w3992:dbl)  [unwired: 2 in]
                    n3058 = Number To Fractional String(number=w3992, precision (6)=i16 9) -> (F-format string=w3990:string)  [unwired: 2 in]
                    n3059 = call "Comma_to_Point.vi"("Lat_A"=w3990) -> ("Saída"=w3989:string)
                  }
                }
                n3060 = global write "Global_Telescopio.vi" "Centragem Via Aquisicao"(FALSE ("Centragem Via Aquisicao")) -> ()
                n3061 = local write "Processa Centragem"(TRUE) -> ()
                n3062 = global write "Global_Telescopio.vi" "NAME OBJETO"(w3985) -> ()
                n3063 = global write "Global_Telescopio.vi" "DEC AQUIS"(w3983) -> ()
                n3064 = global write "Global_Telescopio.vi" "RA AQUIS"(w3984) -> ()
                n3065 = Concatenate Strings(w3985, w3982, w3984, w3982, w3983) -> (w3981:string)
                n3066 = global write "Global_Telescopio.vi" "EPOCH AQUIS"(w3980) -> ()
              }
              frame #2 {
                w3993 = "\t"
                w4008 = FALSE ("use system decimal point (T)")
                w4009 = i16 1 ("precision (6)")
                n3067 = global read "Global_Telescopio.vi" "Right Ascention"() -> (w3999:string)
                n3068 = global read "Global_Telescopio.vi" "Calagem DEC"() -> (w4025:dbl)
                n3069 = global read "Global_Telescopio.vi" "Calagem AH"() -> (w4022:dbl)
                n3070 = global read "Global_Telescopio.vi" "Sideral Time"() -> (w4018:dbl)
                n3071 = global read "Global_Telescopio.vi" "Sideral time"() -> (w3996:string)
                n3072 = global read "Global_Telescopio.vi" "Hour Angle"() -> (w3997:string)
                n3073 = global read "Global_Telescopio.vi" "Declination"() -> (w3998:string)
                n3074 = global read "Global_Telescopio.vi" "TargetDEC"() -> (w4013:dbl)
                n3075 = global read "Global_Telescopio.vi" "TargetRA"() -> (w4012:dbl)
                n3076 = local read "Offset DEC"() -> (w4011:dbl)
                n3077 = local read "Offset RA"() -> (w4010:dbl)
                n3078 = global read "Global_Telescopio.vi" "PosDEC"() -> (w4016:dbl)
                n3079 = global read "Global_Telescopio.vi" "PosAH"() -> (w4019:dbl)
                n3080 = local read "UT"() -> (w3994:string)
                n3081 = Subtract(x=w4018, y=w4019) -> (x-y=w4017:dbl)
                n3082 = call "rad_hms.vi"("TRUE=HORA\nFALSE=GRAU"=TRUE ("TRUE=HORA\nFALSE=GRAU"), "Radiano"=w4012) -> ("Hora/Graus Texto Decimal"=w4006:string)  [unwired: 3 in]
                n3083 = call "rad_hms.vi"("TRUE=HORA\nFALSE=GRAU"=FALSE ("TRUE=HORA\nFALSE=GRAU"), "Radiano"=w4013) -> ("Hora/Graus Texto Decimal"=w4005:string)  [unwired: 3 in]
                n3084 = call "rad_hms.vi"("TRUE=HORA\nFALSE=GRAU"=TRUE ("TRUE=HORA\nFALSE=GRAU"), "Radiano"=w4017) -> ("Hora/Graus Texto Decimal"=w4004:string)  [unwired: 3 in]
                n3085 = call "rad_hms.vi"("TRUE=HORA\nFALSE=GRAU"=FALSE ("TRUE=HORA\nFALSE=GRAU"), "Radiano"=w4016) -> ("Hora/Graus Texto Decimal"=w4003:string)  [unwired: 3 in]
                n3086 = call "rad_hms.vi"("TRUE=HORA\nFALSE=GRAU"=TRUE, "Radiano"=w4022) -> ("Hora/Graus Texto Decimal"=w4002:string)  [unwired: 3 in]
                n3087 = call "rad_hms.vi"("TRUE=HORA\nFALSE=GRAU"=FALSE, "Radiano"=w4025) -> ("Hora/Graus Texto Decimal"=w4007:string)  [unwired: 3 in]
                n3088 = Number To Fractional String(use system decimal point (T)=w4008, number=w4011, precision (6)=w4009) -> (F-format string=w4001:string)  [unwired: 1 in]
                n3089 = Number To Fractional String(use system decimal point (T)=w4008, number=w4010, precision (6)=w4009) -> (F-format string=w4000:string)  [unwired: 1 in]
                n3090 = Concatenate Strings(w4006, w3993, w4005, w3993, w4004, w3993, w4003, w3993, w4002, w3993, w4007, w3993, w4001, w3993, w4000, w3993, w3999, w3993, w3998, w3993, w3997, w3993, w3996, w3993, w3994) -> (w3995:string)
              }
              frame #3 {
                w4027 = TRUE
                w4026 = FALSE
                w4029 = "\t"
                # "MUDANÇA 30-03-2024: Inseridos no LOG  os valores de coordenadas de \ninteresse para um levantamento de erros de apontamento do telescópio."
                n3091 = global read "Global_Telescopio.vi" "PointingModel DEC"() -> (w4051:dbl)
                n3092 = global read "Global_Telescopio.vi" "PointingModel RA"() -> (w4052:dbl)
                n3093 = global read "Global_Telescopio.vi" "Precessed  DEC"() -> (w4053:dbl)
                n3094 = global read "Global_Telescopio.vi" "Calagem DEC"() -> (w4055:dbl)
